vi "Display Test.vi"() -> ()   [LabVIEW 2019]
uses:
  Display/Public/Controls/Size.ctl
  Pixel/Pixel.lvclass
  C:/Users/goo13/Documents/GIT Local/myRIO-Neopixel/Source/RT/Display Element/Display Element.lvclass
  Display Element/Public/Controls/Vector.ctl
  <vilib>/numeric/Random Number (Range) I64.vi
  <vilib>/numeric/Random Number (Range) U64.vi
  <vilib>/numeric/sub_Random U32.vi
  Display/Display.lvclass
  Display Element/Display Element.lvclass
panel:
  in  "Boolean":bool
  out "Frame":u32[][](array[colorbox])
  in  "stop":bool
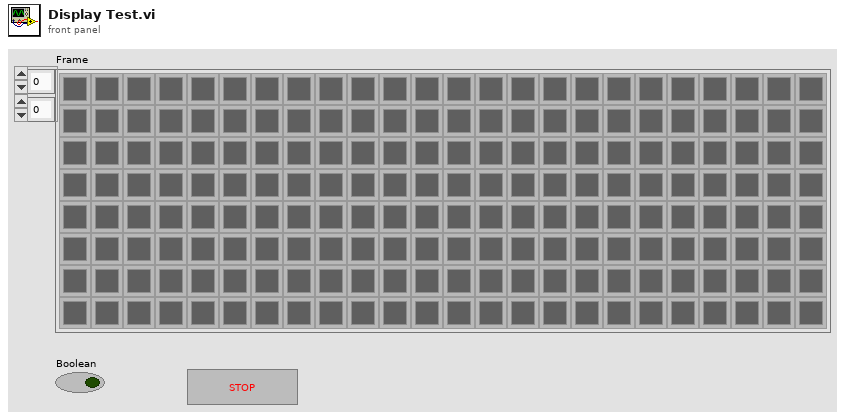
[diagram p1: front panel]
types:
  T1 = typedef "Display.lvclass/Size.ctl" = cluster{"Width":i32, "Height":i32}
  T2 = typedef "Display Element.lvclass/Vector.ctl" = cluster{"X":i32, "Y":i32}
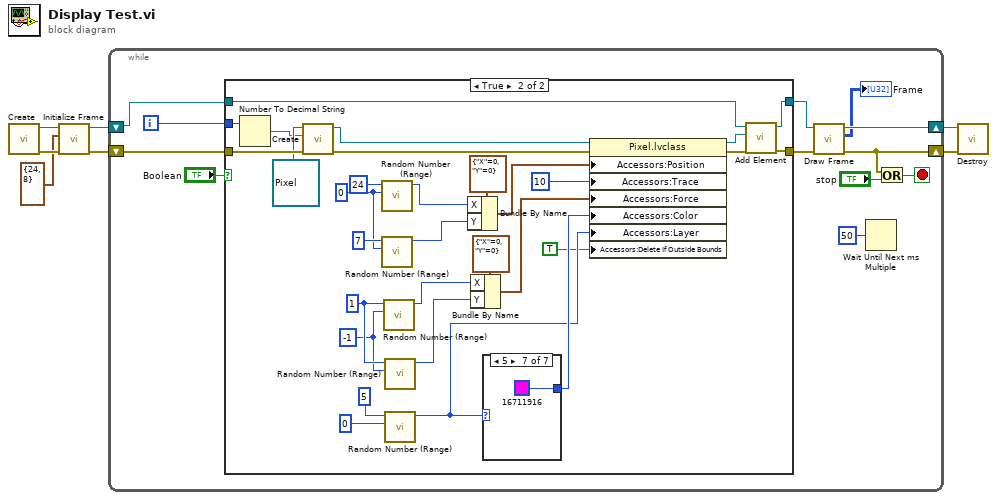
[diagram p0: block diagram]
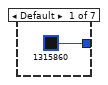
[diagram p3: hidden frame]
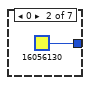
[diagram p4: hidden frame]
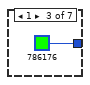
[diagram p5: hidden frame]
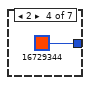
[diagram p6: hidden frame]
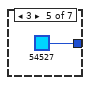
[diagram p7: hidden frame]
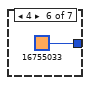
[diagram p8: hidden frame]
diagram:
  n1 = call "Create.vi"() -> ("Error Out"=w4:errorcluster, "Screen Out"=w5:refnum<class "Display.lvclass">)  [unwired: 10 in]
  n2 = call "Initialize Frame.vi"("Error In"=w4, "Size"=T1 {"Width"=24, "Height"=8}, "Display In"=w5) -> ("Error Out"=w1:errorcluster, "Display Out"=w2:refnum<class "Display.lvclass">)  [unwired: 7 in]
  n3 = while {
    shift-right: [w17] -> w6
    shift-left: w1 -> [w14]
    shift-right: [w19] -> w7
    shift-left: w2 -> [w13]
    i -> [w10]
    stop <- w15 stop-if-true
    n4 = case shown="True" "Boolean" {
      tunnel: w14 -> [w20 w51]
      tunnel: w10 -> [_ w49]
      tunnel: w13 -> [w21 w47]
      tunnel: [w21 w46] -> w12
      tunnel: [w20 w45] -> w11
      frame False {
      }
      frame True {
        w27 = i64 -1 ("upper bound (100)")
        w30 = i64 1 ("upper bound (100)")
        w31 = u64 0 ("lower bound (0)")
        n5 = Number To Decimal String(number=w49) -> (decimal integer string=w48:string)  [unwired: 1 in]
        n6 = call-dynamic "Create.vi"("Error In"=w51, "Tag"=w48, "Pixel In"=refnum<class "Pixel.lvclass"> refnum) -> ("Error Out"=w43:errorcluster, "Pixel Out"=w44:refnum<class "Pixel.lvclass">)  [unwired: 7 in]
        n7 = call-poly <vilib>:"Random Number (Range).vi"("lower bound (0)"=w31, "upper bound (100)"=u64 24) -> ("number"=w38:u64)  [unwired: 9 in]
        n8 = call-poly <vilib>:"Random Number (Range).vi"("lower bound (0)"=w31, "upper bound (100)"=u64 7) -> ("number"=w36:u64)  [unwired: 9 in]
        n9 = call-poly <vilib>:"Random Number (Range).vi"("lower bound (-100)"=w27, "upper bound (100)"=w30) -> ("number"=w29:i64)  [unwired: 9 in]
        n10 = call-poly <vilib>:"Random Number (Range).vi"("lower bound (-100)"=w27, "upper bound (100)"=w30) -> ("number"=w28:i64)  [unwired: 9 in]
        n11 = call-poly <vilib>:"Random Number (Range).vi"("lower bound (-100)"=i64 0, "upper bound (100)"=i64 5) -> ("number"=w23:i64)  [unwired: 9 in]
        n12 = Bundle By Name(cluster=T2 {"X"=0, "Y"=0} ("Position"), "X"=w38, "Y"=w36) -> (w35:T2)
        n13 = Bundle By Name(cluster=T2 {"X"=0, "Y"=0} ("Position"), "X"=w29, "Y"=w28) -> (w32:T2)
        n14 = case shown="5" w23 {
          tunnel: [u32 1315860 ("Color") u32 16056130 ("Color") u32 786176 ("Color") u32 16729344 ("Color") u32 54527 ("Color") u32 16755033 ("Color") u32 16711916 ("Color")] -> w24
          frame Default {
          }
          frame 0 {
          }
          frame 1 {
          }
          frame 2 {
          }
          frame 3 {
          }
          frame 4 {
          }
          frame 5 {
          }
        }
        n15 = property class="Pixel.lvclass"(reference=w44, error in=w43, "Accessors:Position"=w35, "Accessors:Trace"=10 ("Trace"), "Accessors:Force"=w32, "Accessors:Color"=w24, "Accessors:Layer"=w23, "Accessors:Delete If Outside Bounds"=TRUE ("Delete If Outside Bounds")) -> (reference out=w42:refnum<class "Pixel.lvclass">, error out=w41:errorcluster)
        n16 = call "Add Element.vi"("Error In"=w41, "New Element"=w42, "Display In"=w47) -> ("Error Out"=w45:errorcluster, "Display Out"=w46:refnum<class "Display.lvclass">)  [unwired: 7 in]
      }
    }
    n17 = call "Draw Frame.vi"("Error In"=w11, "Display In"=w12) -> ("Error Out"=w17:errorcluster, "Frame"=→"Frame":u32[][], "Display Out"=w19:refnum<class "Display.lvclass">)  [unwired: 7 in]
    n18 = Wait Until Next ms Multiple(millisecond multiple=u32 50) -> ()  [unwired: 1 out]
    n19 = Or(x=w17, y="stop") -> (x .or. y?=w15:bool)
  }
  n20 = call "Destroy.vi"("Error In"=w6, "Display In"=w7) -> ()  [unwired: 9 in, 1 out]
